vi "CmdToDb.vi"(0 "reference in":refnum<class "Device.lvclass">, 5 "CMD":string=".ST", 7 "Value":string, 11 "error in (no error)":errorcluster) -> (4 "reference out":refnum<class "Device.lvclass">, 15 "error out":errorcluster)   [LabVIEW 2019, in "Device.lvclass"]
uses:
  Device.lvclass
  D:/GIT H4000/H4000/src/Proccess_class/Proccess.lvclass
  Proccess_class/Proccess.lvclass/Proccess.ctl
  Logger_class/EventType.ctl
  Logger_class/EventData.ctl
  TypeDef/AlarmType.ctl
  Logger_class/Logger.lvclass
  Proccess_class/Proccess.lvclass
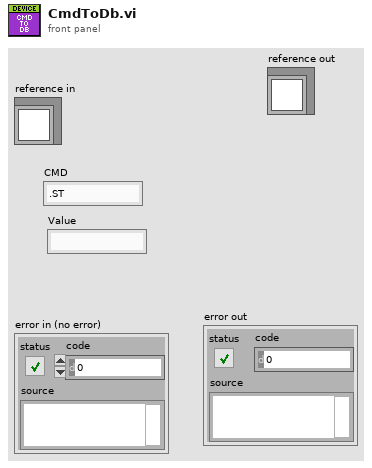
[diagram p1: front panel]
types:
  T1 = typedef "Logger.lvclass/EventType.ctl" = enum16{"DI_LO", "DI_HI", "DO_LO", "DO_HI", "DA_LO", "DA_HI", "AA_LO", "AA_HI", "CMD", "ERR", "ST"}
  T2 = typedef "Logger.lvclass/EventData.ctl" = cluster{"obj_tag":string, "event_tag":string, "Description":string, "EVENT TYPE":T1, "ALARM TYPE":T3, "Value DBL":dbl, "Value INT":i32, "Value STR":string, "Time Stamp":timestamp}
  T3 = typedef "AlarmType.ctl" = enum16{"Normal", "Warning", "Alarm"}
  T4 = typedef "Proccess.lvclass/TAGs.ctl" = cluster{"TAG":string, "PTAG":string, "DESC":string}
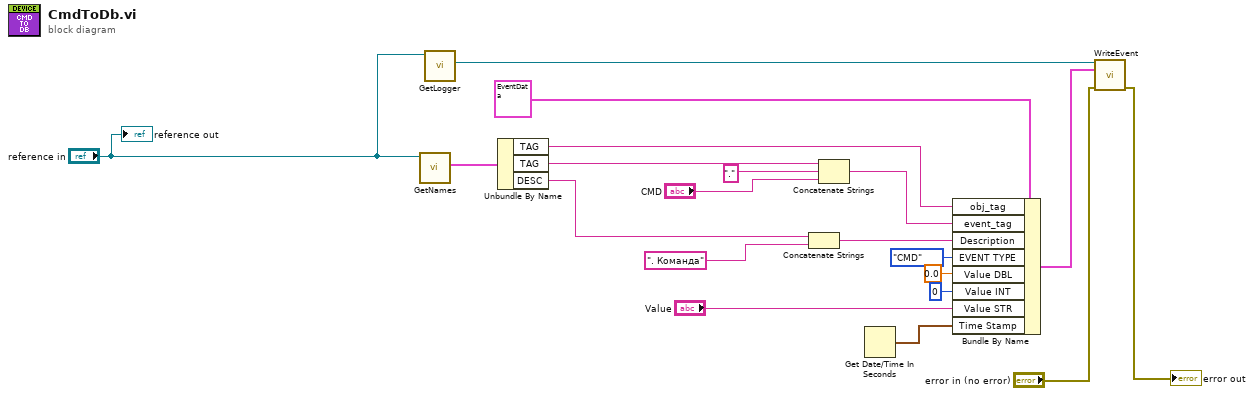
[diagram p0: block diagram]
diagram:
  n1 = call "GetNames.vi"("Proccess in"="reference in") -> ("Tags"=w11:T4)  [unwired: 10 in]
  n2 = call "GetLogger.vi"("Proccess in"="reference in") -> ("Logger"=w12:refnum<class "Logger.lvclass">)  [unwired: 10 in]
  n3 = Unbundle By Name(w11) -> ("TAG"=w10:string, "TAG"=w9:string, "DESC"=w8:string)
  n4 = Concatenate Strings(w8, ". Команда" ("string")) -> (w5:string)
  n5 = Concatenate Strings(w9, "." ("string"), "CMD") -> (w14:string)
  n6 = Get Date/Time In Seconds() -> (seconds since 1Jan1904=w7:timestamp)
  n7 = Bundle By Name(cluster=T2 {"obj_tag"="", "event_tag"="", "Description"="", "EVENT TYPE"=enum."DA_LO", "ALARM TYPE"=enum."Alarm", "Value DBL"=0.0, "Value INT"=0, "Value STR"="", "Time Stamp"=timestamp(0 s since 1904-01-01)} ("Event"), "obj_tag"=w10, "event_tag"=w14, "Description"=w5, "EVENT TYPE"=EventType."CMD", "Value DBL"=0.0, "Value INT"=0, "Value STR"="Value", "Time Stamp"=w7) -> (w16:T2)
  n8 = call "WriteEvent.vi"("reference in"=w12, "Event"=w16, "error in (no error)"="error in (no error)") -> ("error out"=→"error out":errorcluster)  [unwired: 11 in, 1 out]
  "reference out" <- "reference in"
